vi "Process DS402 SM.vi"(0 "DS402 IOV in":T6, 1 "R/W Case":T1, 5 "I/O Output Data In":T5 {"BD Refs"."Data Reference" format="%.0x"}, 9 "I/O Input Data In":T2 {"BD Refs"."Data Reference" format="%.0x"}, 11 "error in (no error)":errorcluster) -> (4 "DS402 IOV out":T6, 6 "I/O Output Data Out":T5 {"BD Refs"."Data Reference" format="%.0x"}, 10 "I/O Input Data Out":T2 {"BD Refs"."Data Reference" format="%.0x"}, 15 "error out":errorcluster)   [LabVIEW 2016, in "Scan Engine Custom Device.lvlib"]
uses:
  Scan Engine Custom Device.lvlib
  Type Defs/DS402 Drive ECAT Slave Action IOV Cluster.ctl
  Library/controls/state.ctl
  Type Defs/Output Data.ctl
  <vilib>/NI Veristand/Custom Device API/Block Data Reference.ctl
  <vilib>/NI Veristand/Custom Device API/Data Reference.ctl
  Type Defs/Input Data.ctl
  Type Defs/RW Case.ctl
  Library/controls/control word commands.ctl
  Library/DS402.lvlib
  <vilib>/NI/syslog/_subVIs/TypeDefs/syslog_severity_codes.ctl
  <vilib>/NI Veristand/Custom Device API/Custom Device API.lvlib
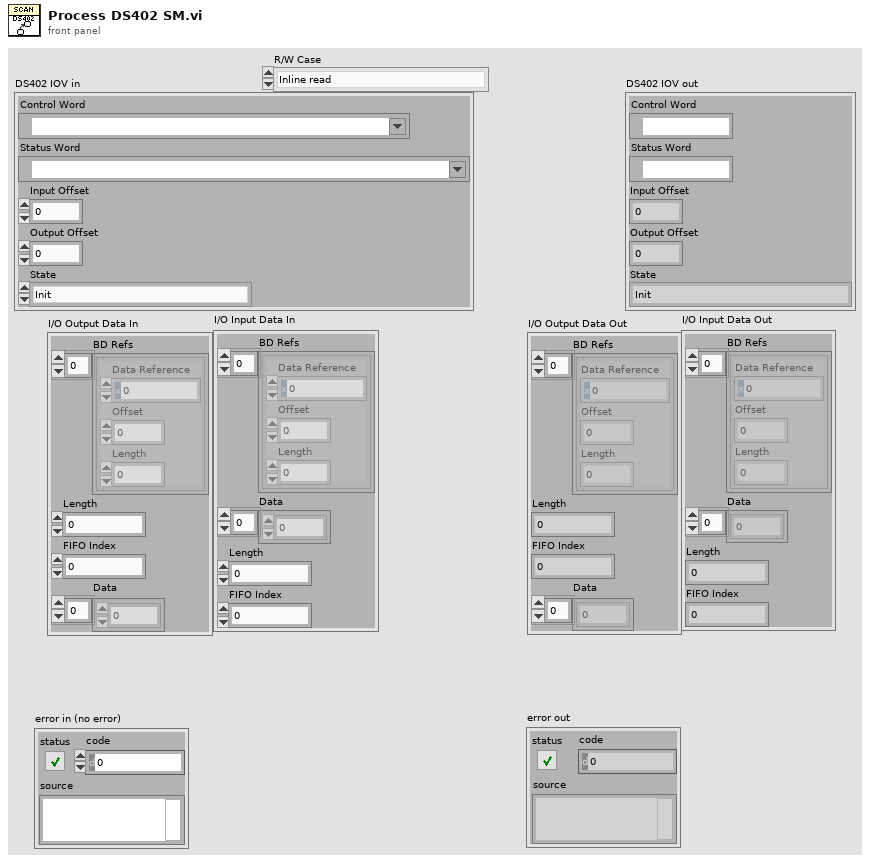
[diagram p1: front panel]
types:
  T1 = typedef "Scan Engine Custom Device.lvlib/RW Case.ctl" = enum16{"Inline read", "Inline write", "Async - Inline loop read", "Async - Inline loop write", "Async loop (read/write)"}
  T2 = typedef "Scan Engine Custom Device.lvlib/Input Data.ctl" = cluster{"BD Refs":T3[], "Data":dbl[], "Length":i32, "FIFO Index":i32}
  T3 = typedef "Custom Device API.lvlib/Block Data Reference.ctl" = cluster{"Data Reference":T4, "Offset":u64, "Length":u64}
  T4 = typedef "Custom Device API.lvlib/Data Reference.ctl" = i32
  T5 = typedef "Scan Engine Custom Device.lvlib/Output Data.ctl" = cluster{"BD Refs":T3[], "Length":i32, "FIFO Index":i32, "Data":dbl[]}
  T6 = typedef "Scan Engine Custom Device.lvlib/DS402 Drive ECAT Slave Action IOV Cluster.ctl" = cluster{"Control Word":refnum<k21>, "Status Word":refnum<k21>, "Input Offset":i32, "Output Offset":i32, "State":T7}
  T7 = typedef "Scan Engine Custom Device.lvlib/DS402.lvlib/state.ctl" = enum16{"Init", "Not Ready to Switch On", "Read Status Word", "Switch on disabled", "Ready to switch on", "Switched on", "Operation enabled", "Fault", "Fault reaction active", "Quick stop active", "Shutdown - Bad State", "Shutdown - Error", "Shutdown - Normal", "Shutdown - Fault"}
  T8 = typedef "syslog_severity_codes.ctl" = enum16{"emergency", "alert", "critical", "error", "warning", "notice", "info", "debug"}
  T9 = typedef "Scan Engine Custom Device.lvlib/DS402.lvlib/control word commands.ctl" = u16
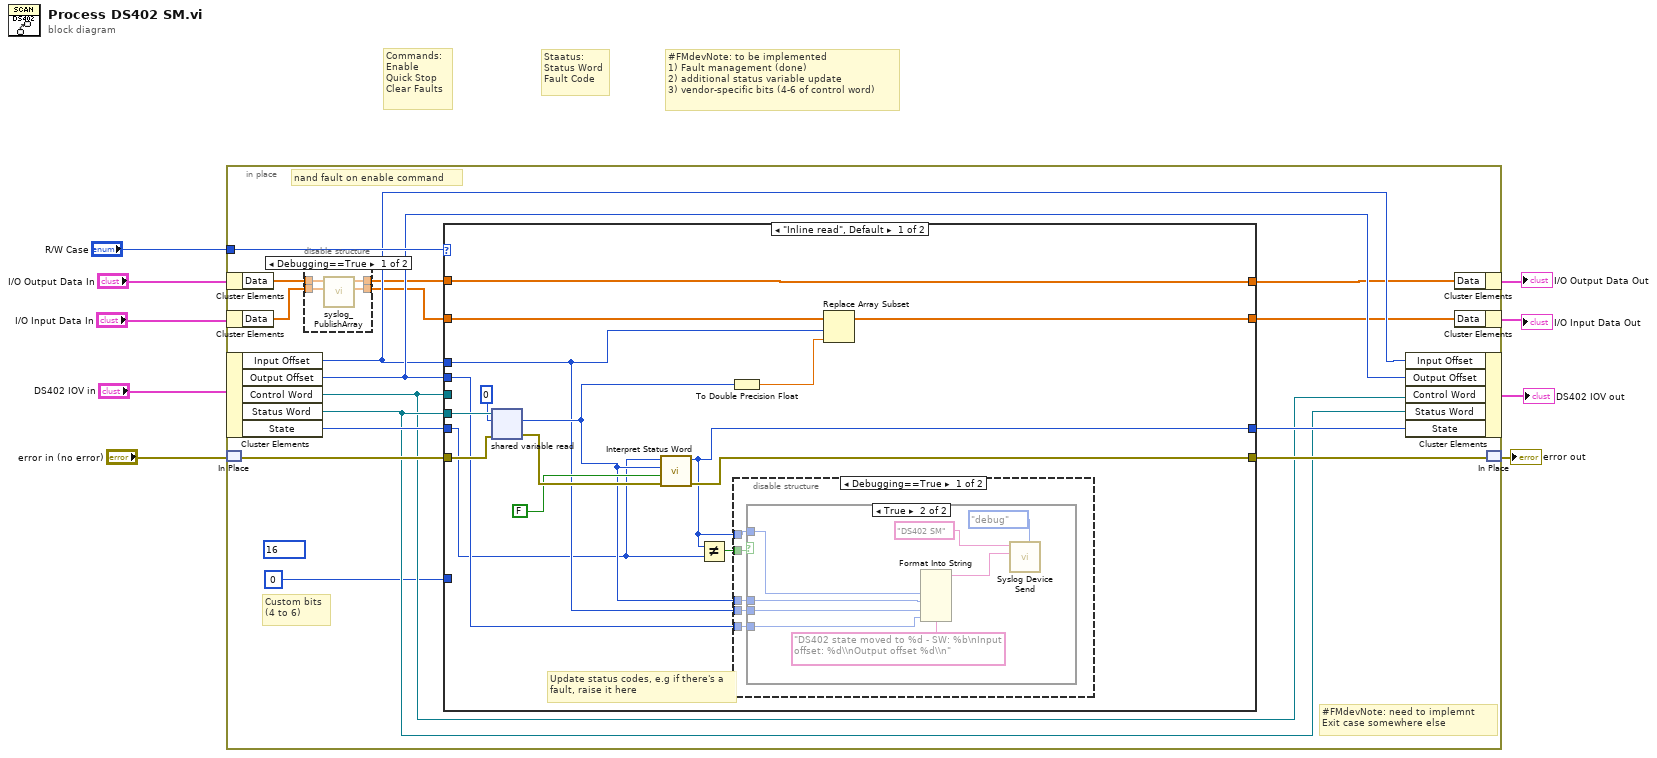
[diagram p0: block diagram]
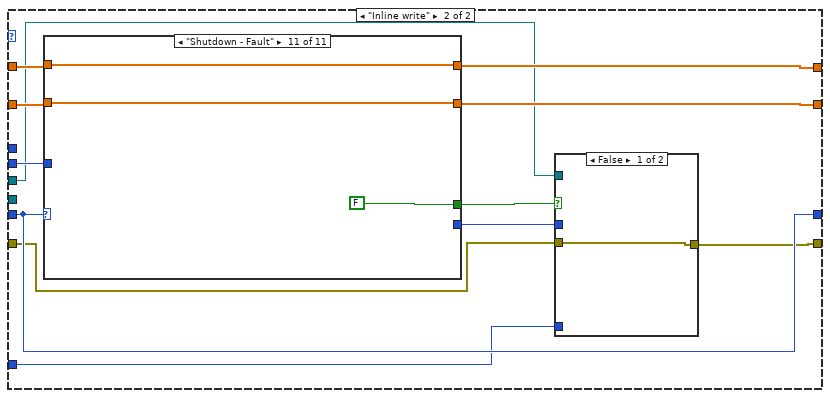
[diagram p5: hidden frame]
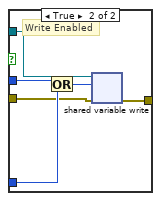
[diagram p6: hidden frame]
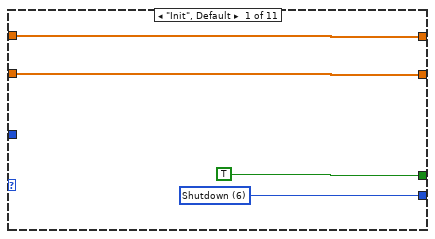
[diagram p7: hidden frame]
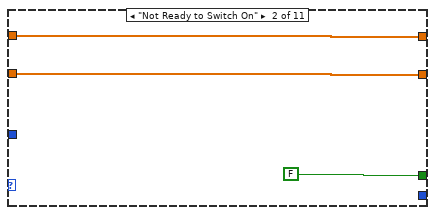
[diagram p8: hidden frame]
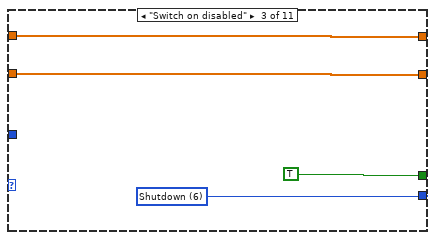
[diagram p9: hidden frame]
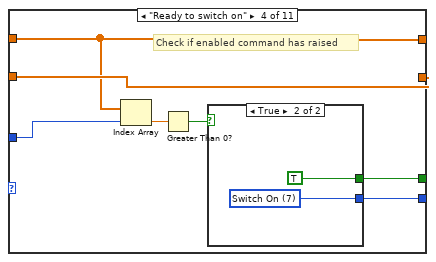
[diagram p10: hidden frame]
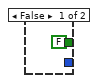
[diagram p11: hidden frame]
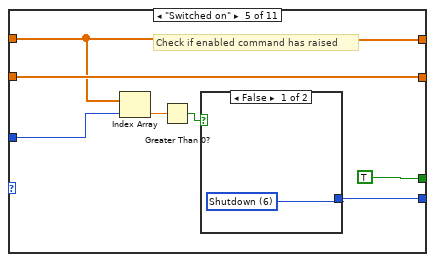
[diagram p12: hidden frame]
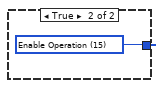
[diagram p13: hidden frame]
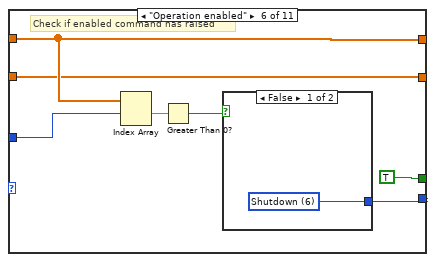
[diagram p14: hidden frame]
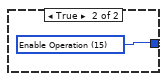
[diagram p15: hidden frame]
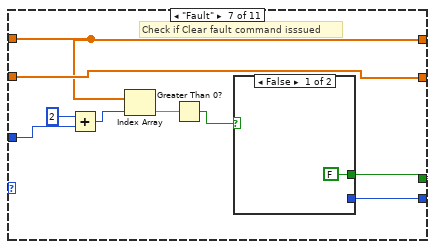
[diagram p16: hidden frame]
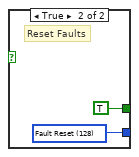
[diagram p17: hidden frame]
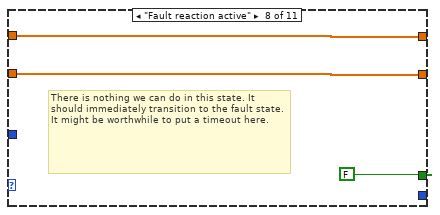
[diagram p18: hidden frame]
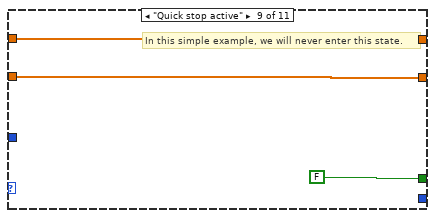
[diagram p19: hidden frame]
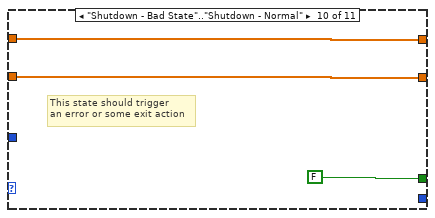
[diagram p20: hidden frame]
diagram:
  # "Staatus:\nStatus Word\nFault Code"
  # "Commands:\nEnable\nQuick Stop\nClear Faults"
  # "#FMdevNote: to be implemented\n1) Fault management (done)\n2) additional status variable update\n3) vendor-specific bits (4-6 of control word)"
  n1 = in-place {
    in-place-border: "R/W Case" -> [w25]
    (unwired) u16 16
    # "Custom bits\n(4 to 6)"
    # "nand fault on enable command"
    # "#FMdevNote: need to implemnt\nExit case somewhere else"
    n2 = in-place-cluster #1("I/O Output Data In") -> ("Data"=w14:dbl[])
    n3 = in-place-cluster #2("I/O Input Data In") -> ("Data"=w13:dbl[])
    n4 = in-place-cluster #3("DS402 IOV in") -> ("Input Offset"=w19:i32, "Output Offset"=w20:i32, "Control Word"=w15:refnum<k21>, "Status Word"=w16:refnum<k21>, "State"=w24:T7)
    n5 = in-place-match #4("error in (no error)") -> (w23:errorcluster)
    n6 = disable-structure shown="Debugging==True" {
      disable-tunnel: w14 -> [w26 w31]
      disable-tunnel: w13 -> [w29 w30]
      disable-tunnel: [w28 w31] -> w12
      disable-tunnel: [w27 w30] -> w11
      frame condition #0 {
        n7 = call "syslog_PublishArray.vi"("Input Array In"=w29, "Output Array In"=w26) -> ("Input Array Out"=w27:dbl[], "Output Array Out"=w28:dbl[])  [unwired: 8 in]
      }
      frame condition #1 (active) {
      }
    }
    n8 = case shown="\"Inline read\", Default" w25 {
      tunnel: w16 -> [w45 _]
      tunnel: w24 -> [w32 w67]
      tunnel: w23 -> [w44 w61]
      tunnel: [w43 w63] -> w22
      tunnel: w11 -> [w42 w71]
      tunnel: w19 -> [w34 _]
      tunnel: [w40 w69] -> w17
      tunnel: [w36 w67] -> w21
      tunnel: w20 -> [w33 w68]
      tunnel: [w39 w70] -> w18
      tunnel: w12 -> [w39 w72]
      tunnel: w15 -> [_ w66]
      tunnel: u16 0 -> [_ w65]
      frame "Inline read", Default {
        # "Update status codes, e.g if there's a\nfault, raise it here"
        n9 = shared-variable-read(w45, w44, u16 0 ("data type")) -> (w47:errorcluster, w35:u16)  [unwired: 2 out]
        n10 = call "Interpret Status Word.vi"("error in (no error)"=w47, "Exit"=FALSE, "Status Word In"=w35, "State In"=w32) -> ("error out"=w43:errorcluster, "State Out"=w36:T7)  [unwired: 6 in]
        n11 = Not Equal?(x=w36, y=w32) -> (x != y?=w37:bool)
        n12 = To Double Precision Float(number=w35) -> (double precision float=w41:dbl)
        n13 = disable-structure shown="Debugging==True" {
          disable-tunnel: w37 -> [w52 _]
          disable-tunnel: w36 -> [w51 _]
          disable-tunnel: w35 -> [w50 _]
          disable-tunnel: w34 -> [w49 _]
          disable-tunnel: w33 -> [w48 _]
          frame condition #0 {
            n14 = case shown="True" w52 {
              tunnel: w51 -> [_ w57]
              tunnel: w50 -> [_ w55]
              tunnel: w49 -> [_ w54]
              tunnel: w48 -> [_ w53]
              frame False {
              }
              frame True {
                n15 = Format Into String(format string="DS402 state moved to %d - SW: %b\nInput offset: %d\\nOutput offset %d\\n", w57, w55, w54, w53) -> (resulting string=w58:string)  [unwired: 2 in, 1 out]
                n16 = call <vilib>:"Syslog Device Send.vi"("Severity Code (error)"=syslog_severity_codes."debug", "Message Content"=w58, "Message Tag"="DS402 SM") -> ()  [unwired: 7 in, 2 out]
              }
            }
          }
          frame condition #1 (active) {
          }
        }
        n17 = Replace Array Subset(array=w42, new element=w41, index=w34) -> (w40:dbl[])
      }
      frame "Inline write" {
        n18 = case shown="\"Shutdown - Fault\"" w67 {
          tunnel: w71 -> [w83 w86 w89 w97 w107 w115 w127 w133 w136 w139 w141]
          tunnel: w72 -> [w82 w85 w90 w96 w106 w116 w126 w132 w135 w138 w142]
          tunnel: [w82 w85 w90 w96 w106 w116 w126 w132 w135 w138 w142] -> w70
          tunnel: [w83 w86 w89 w97 w107 w115 w127 w133 w136 w139 w141] -> w69
          tunnel: w68 -> [_ _ _ w95 w105 w112 w125 _ _ _ _]
          tunnel: [w80 _ w88 w92 w102 w111 w120 _ _ _ _] -> w64
          tunnel: [TRUE FALSE TRUE w91 TRUE TRUE w119 FALSE FALSE FALSE FALSE] -> w62
          frame "Init", Default {
            w80 = T9 6 items=["Shutdown"=6, "Disable Voltage"=0, "Fault Reset"=128, "Quick Stop"=2, "Enable Operation"=15, "Switch On"=7] ("Ring")
          }
          frame "Not Ready to Switch On" {
          }
          frame "Switch on disabled" {
            w88 = T9 6 items=["Shutdown"=6, "Disable Voltage"=0, "Fault Reset"=128, "Quick Stop"=2, "Enable Operation"=15, "Switch On"=7] ("Ring")
          }
          frame "Ready to switch on" {
            # "Check if enabled command has raised"
            n19 = Index Array(array=w96, index=w95) -> (element=w94:dbl)
            n20 = Greater Than 0?(x=w94) -> (x > 0?=w93:bool)
            n21 = case shown="True" w93 {
              tunnel: [_ w100] -> w92
              tunnel: [FALSE TRUE] -> w91
              frame False {
              }
              frame True {
                w100 = T9 7 items=["Shutdown"=6, "Disable Voltage"=0, "Fault Reset"=128, "Quick Stop"=2, "Enable Operation"=15, "Switch On"=7] ("Ring")
              }
            }
          }
          frame "Switched on" {
            # "Check if enabled command has raised"
            n22 = Index Array(array=w106, index=w105) -> (element=w104:dbl)
            n23 = Greater Than 0?(x=w104) -> (x > 0?=w103:bool)
            n24 = case shown="False" w103 {
              tunnel: [w108 w109] -> w102
              frame False {
                w108 = T9 6 items=["Shutdown"=6, "Disable Voltage"=0, "Fault Reset"=128, "Quick Stop"=2, "Enable Operation"=15, "Switch On"=7] ("Ring")
              }
              frame True {
                w109 = T9 15 items=["Shutdown"=6, "Disable Voltage"=0, "Fault Reset"=128, "Quick Stop"=2, "Enable Operation"=15, "Switch On"=7] ("Ring")
              }
            }
          }
          frame "Operation enabled" {
            # "Check if enabled command has raised"
            n25 = Index Array(array=w116, index #1=w112) -> (element #1=w114:dbl)  [unwired: 1 in, 1 out]
            n26 = Greater Than 0?(x=w114) -> (x > 0?=w113:bool)
            n27 = case shown="False" w113 {
              tunnel: [w117 w118] -> w111
              frame False {
                w117 = T9 6 items=["Shutdown"=6, "Disable Voltage"=0, "Fault Reset"=128, "Quick Stop"=2, "Enable Operation"=15, "Switch On"=7] ("Ring")
              }
              frame True {
                w118 = T9 15 items=["Shutdown"=6, "Disable Voltage"=0, "Fault Reset"=128, "Quick Stop"=2, "Enable Operation"=15, "Switch On"=7] ("Ring")
              }
            }
          }
          frame "Fault" {
            # "Check if Clear fault command isssued"
            n28 = Add(x=2, y=w125) -> (x+y=w124:i32)
            n29 = Index Array(array=w126, index=w124) -> (element=w123:dbl)
            n30 = Greater Than 0?(x=w123) -> (x > 0?=w122:bool)
            n31 = case shown="False" w122 {
              tunnel: [_ w130] -> w120
              tunnel: [FALSE TRUE] -> w119
              frame False {
              }
              frame True {
                w130 = T9 128 items=["Shutdown"=6, "Disable Voltage"=0, "Fault Reset"=128, "Quick Stop"=2, "Enable Operation"=15, "Switch On"=7] ("Ring")
                # "Reset Faults"
              }
            }
          }
          frame "Fault reaction active" {
            # "There is nothing we can do in this state. It should immediately transition to the fault state.\nIt might be worthwhile to put a timeout here."
          }
          frame "Quick stop active" {
            # "In this simple example, we will never enter this state."
          }
          frame "Shutdown - Bad State".."Shutdown - Normal" {
            # "This state should trigger \nan error or some exit action"
          }
          frame "Shutdown - Fault" {
          }
        }
        n32 = case shown="False" w62 {
          tunnel: w66 -> [_ w79]
          tunnel: w65 -> [_ w78]
          tunnel: w64 -> [_ w76]
          tunnel: [w73 w75] -> w63
          tunnel: w61 -> [w73 w74]
          frame False {
          }
          frame True {
            # "Write Enabled"
            n33 = Or(x=w76, y=w78) -> (x .or. y?=w77:T9)
            n34 = shared-variable-write(w79, w74, w77) -> (w75:errorcluster)  [unwired: 1 out]
          }
        }
      }
    }
    n35 = in-place-cluster #3("Input Offset"=w19, "Output Offset"=w20, "Control Word"=w15, "Status Word"=w16, "State"=w21) -> (→"DS402 IOV out":T6)
    n36 = in-place-cluster #1("Data"=w18) -> (→"I/O Output Data Out":T5)
    n37 = in-place-cluster #2("Data"=w17) -> (→"I/O Input Data Out":T2)
    n38 = in-place-match #4(w22) -> (→"error out":errorcluster)
  }
